vi "Temperature Warnings.vi"(8 "Error In":errorcluster, 11 "Weather Data In":T1={"Current Temperature"=0.0, "Max Temperature"=0.0, "Min Temperature"=0.0, "Temperature Warning?"=FALSE, "Temperature Warning Text"="No Warning"}) -> (0 "Error Out":errorcluster, 3 "Weather Data Out":T1={"Current Temperature"=0.0, "Max Temperature"=0.0, "Min Temperature"=0.0, "Temperature Warning?"=FALSE, "Temperature Warning Text"="No Warning"})   [LabVIEW 2022 SP3]
doc: "This VI is used to determine temperature warning information based on the current temperature and limit settings."
uses:
  Weather Data.ctl
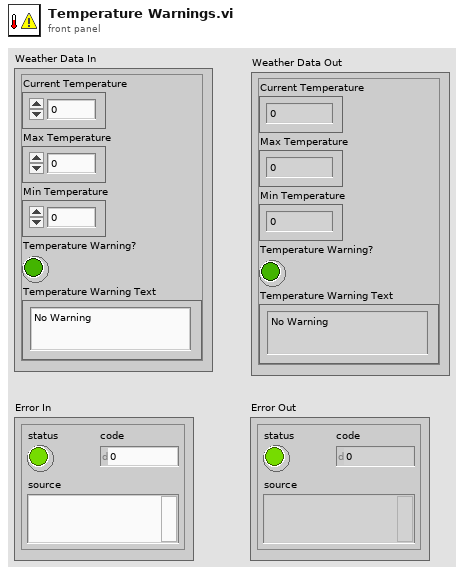
[diagram p1: front panel]
types:
  T1 = typedef "Weather Data.ctl" = cluster{"Current Temperature":dbl, "Max Temperature":dbl, "Min Temperature":dbl, "Temperature Warning?":bool, "Temperature Warning Text":string}
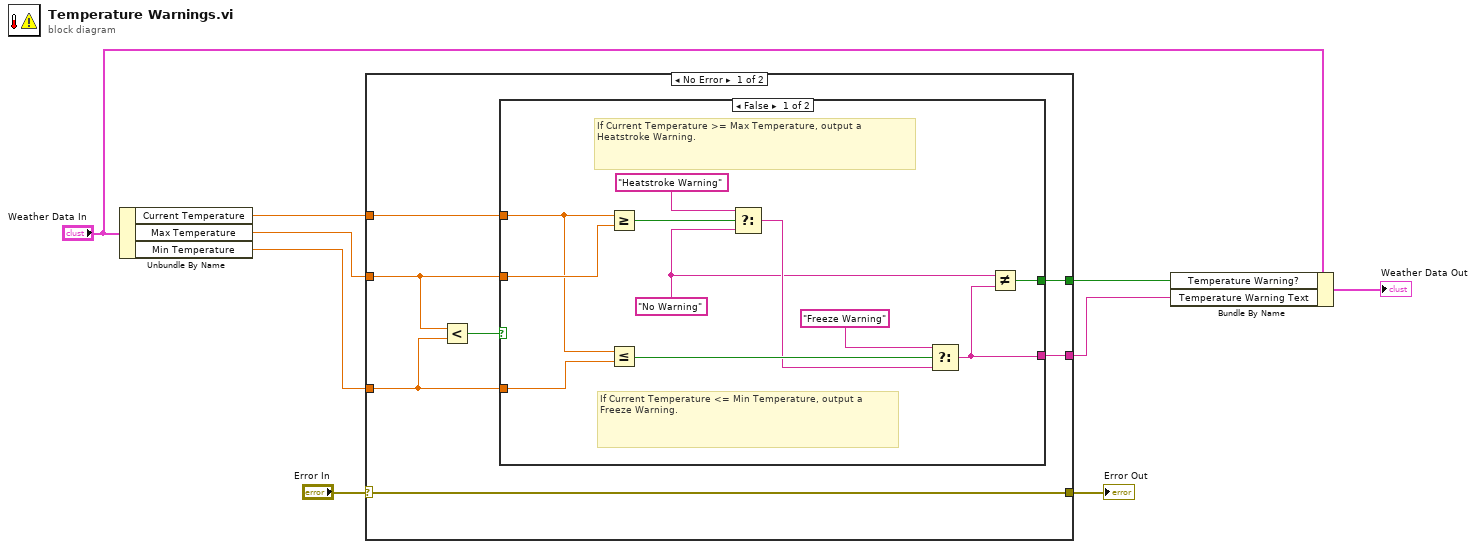
[diagram p0: block diagram]
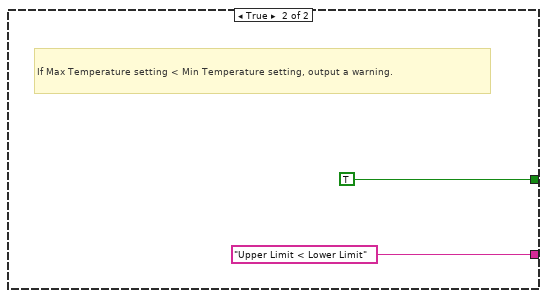
[diagram p2: hidden frame]
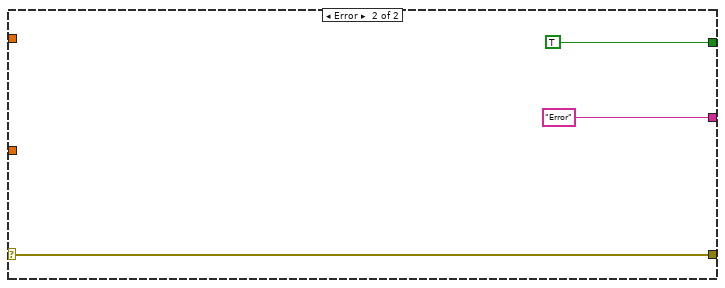
[diagram p3: hidden frame]
diagram:
  n1 = Unbundle By Name("Weather Data In") -> ("Current Temperature"=w7:dbl, "Max Temperature"=w6:dbl, "Min Temperature"=w5:dbl)
  n2 = case shown="No Error" "Error In" {
    selector: "Error In" -> [w14 w32]
    tunnel: [w16 "Error" ("f")] -> w4
    tunnel: [w15 TRUE] -> w3
    tunnel: [w14 w32] -> w8
    tunnel: w5 -> [w11 _]
    tunnel: w7 -> [w13 _]
    tunnel: w6 -> [w12 _]
    frame No Error {
      n3 = Less?(x=w12, y=w11) -> (x < y?=w10:bool)
      n4 = case shown="False" w10 {
        tunnel: [w17 "Upper Limit < Lower Limit" ("f")] -> w16
        tunnel: [w27 TRUE] -> w15
        tunnel: w12 -> [w26 _]
        tunnel: w11 -> [w23 _]
        tunnel: w13 -> [w19 _]
        frame False {
          w18 = "No Warning" ("f")
          # "If Current Temperature <= Min Temperature, output a Freeze Warning."
          # "If Current Temperature >= Max Temperature, output a Heatstroke Warning."
          n5 = Greater Or Equal?(x=w19, y=w26) -> (x >= y?=w25:bool)
          n6 = Less Or Equal?(x=w19, y=w23) -> (x <= y?=w21:bool)
          n7 = Select(t="Heatstroke Warning", s=w25, f=w18) -> (s? t:f=w20:string)
          n8 = Select(t="Freeze Warning", s=w21, f=w20) -> (s? t:f=w17:string)
          n9 = Not Equal?(x=w18, y=w17) -> (x != y?=w27:bool)
        }
        frame True {
          # "If Max Temperature setting < Min Temperature setting, output a warning."
        }
      }
    }
    frame Error {
    }
  }
  "Error Out" <- w8
  n10 = Bundle By Name(cluster="Weather Data In", "Temperature Warning?"=w3, "Temperature Warning Text"=w4) -> (→"Weather Data Out":T1)
